vi "get Rmb User.vi"(5 "[User] Cfg File in":refnum<class "[User] Cfg File.lvclass">) -> (2 "rmb user":bool)   [LabVIEW 2020, in "[User] Cfg File.lvclass"]
uses:
  [User] Cfg File.lvclass
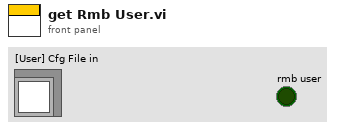
[diagram p1: front panel]
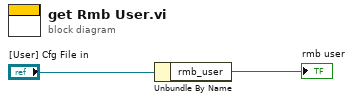
[diagram p0: block diagram]
diagram:
  n1 = Unbundle By Name("[User] Cfg File in") -> ("rmb_user"=→"rmb user":bool)
